vi "ZBX IO DB1.vi"(11 "request":T2) -> (3 "response":T1)   [LabVIEW 2023]
doc: "Does the actual IO for requests/responses to daugtherbord 1.\nNote: Put only <strong>one>/strong> instance of this VI in your FPGA. When multiple requests are send to the daugtherboard use the arbiter VI."
uses:
  <instrlib>/niUSRP/Reference FPGA/ZBX Control/ZBX IO Response.ctl
  <vilib>/eio/EIONode/EIONode.xnode
  <vilib>/rvi/eio/common/nirviEmuTemplateMethod_errors.vi
  <instrlib>/niUSRP/Reference FPGA/ZBX Control/ZBX IO Request.ctl
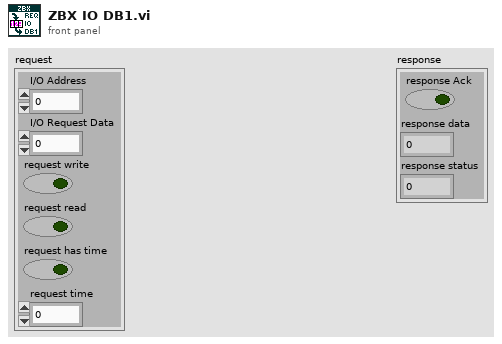
[diagram p1: front panel]
types:
  T1 = typedef "ZBX IO Response.ctl" = cluster{"response Ack":bool, "response data":u32, "response status":fxp<+,2,2>}
  T2 = typedef "ZBX IO Request.ctl" = cluster{"I/O Address":fxp<+,20,20>, "I/O Request Data":u32, "request write":bool, "request read":bool, "request has time":bool, "request time":u64}
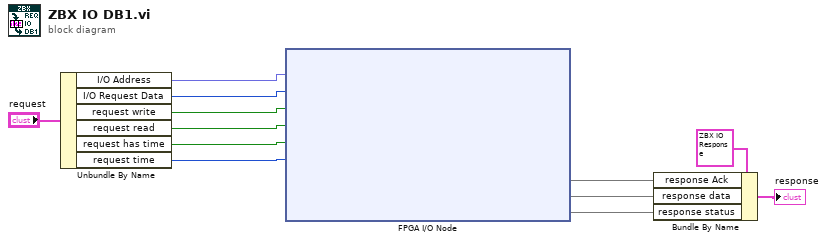
[diagram p0: block diagram]
diagram:
  n1 = Unbundle By Name("request") -> ("I/O Address"=w12:fxp<+,20,20>, "I/O Request Data"=w11:u32, "request write"=w10:bool, "request read"=w9:bool, "request has time"=w8:bool, "request time"=w7:u64)
  n2 = xnode "FPGA I/O Node"("Daughterboard 1\\DBoardCtrlPortReqAddr"=w12, "Daughterboard 1\\DBoardCtrlPortReqData"=w11, "Daughterboard 1\\DBoardCtrlPortReqWr"=w10, "Daughterboard 1\\DBoardCtrlPortReqRd"=w9, "Daughterboard 1\\DBoardCtrlPortReqHasTime"=w8, "Daughterboard 1\\DBoardCtrlPortReqTime"=w7) -> ("Daughterboard 1\\DBoardCtrlPortRespAck"=w3, "Daughterboard 1\\DBoardCtrlPortRespData"=w2, "Daughterboard 1\\DBoardCtrlPortRespStatus"=w1)  [unwired: 9 in, 9 out]
  n3 = Bundle By Name(cluster=T1 {"response Ack"=FALSE, "response data"=0, "response status"=0.0} ("Cluster"), "response Ack"=w3, "response data"=w2, "response status"=w1) -> (→"response":T1)
